vi "Handle Command.vi"(8 "error in (no error)":errorcluster, 10 "CMD in":refnum<class "Set Write Ringdowns CMD.lvclass">, 11 "Object In":refnum<class>) -> (0 "error out":errorcluster, 1 "Command Successful?":bool, 2 "CMD out":refnum<class "Set Write Ringdowns CMD.lvclass">, 3 "Object Out":refnum<class>)   [LabVIEW 2014, in "eCRDS Library.lvlib" / "Set Write Ringdowns CMD.lvclass"]
doc: "This VI will contain the code used to actually execute the request. If the request is successful, this will be indicated by the boolean output <b>Command Successful?</b>. The boolean output can then be used by the <b>Command Reply</b> which sends a reply if the reply queue is valid."
uses:
  Set Write Ringdowns CMD.lvclass
  reusable/CRDS/Main/CRDS.lvclass
  reusable/CRDS/Data/Main/CRDS Data.lvclass
  reusable/Instrument/Instrument.lvclass/Instrument.ctl
  Set Write Ringdowns CMD.lvclass/Set Write Ringdowns CMD.ctl
  reusable/CRDS/Cell/CRDS Cell.lvclass/CRDS Cell.ctl
  reusable/CRDS/Data/Cell/CRDS Cell Data.lvclass/CRDS Cell Data.ctl
  reusable/CRDS/Cell/Read Data.vi
  reusable/CRDS/Data/Cell/Write Write RD_.vi
  reusable/CRDS/Cell/Write Data.vi
  reusable/Instrument/Read Data.vi
  reusable/Instrument/Read Log Session.vi
  reusable/Instrument/Write Data.vi
  reusable/CRDS/Main/Read Cells.vi
  reusable/CRDS/Data/Main/Read CellData.vi
  reusable/CRDS/Data/Main/Write CellData.vi
  reusable/CRDS/Main/Write Cells.vi
  reusable/Data/Data.lvclass
  reusable/CRDS/Cell/CRDS Cell.lvclass
  <userlib>/_Session Fwk/Session - Root.lvclass
  reusable/CRDS/Data/Cell/CRDS Cell Data.lvclass
  reusable/Session APIs/Session Log/System Log.lvclass
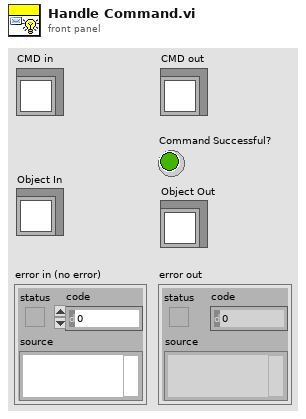
[diagram p1: front panel]
types:
  T1 = typedef "Session - Root.lvclass/Session Handle.ctl" = refnum<data-value>
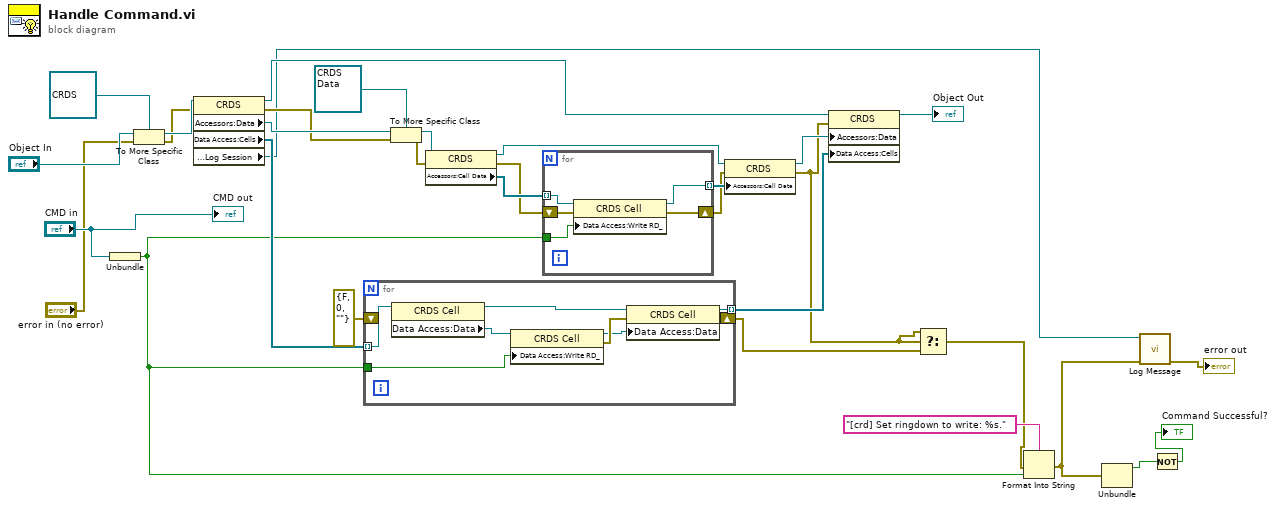
[diagram p0: block diagram]
diagram:
  n1 = Unbundle("CMD in") -> (w6:bool)
  n2 = To More Specific Class(target class=refnum<class "CRDS.lvclass"> refnum ("CRDS Lib.lvlib:CRDS"), reference="Object In", error in="error in (no error)") -> (specific class reference=w30:refnum<class "CRDS.lvclass">, error out=w16:errorcluster)
  n3 = property class="CRDS"(reference=w30, error in=w16) -> (reference out=w21:refnum<class "CRDS.lvclass">, error out=w15:errorcluster, "Accessors:Data"=w29:refnum<class "Data.lvclass">, "Data Access:Cells"=w24:refnum<class "CRDS Cell.lvclass">[], "Accessors:Log Session"=w8:T1)
  n4 = for {
    tunnel: w6 -> [w40]
    tunnel: w24 -> [w39] mode=indexing
    tunnel: [w34] -> w19 mode=indexing
    shift-right: [w33] -> w9
    shift-left: errorcluster {"status"=FALSE, "code"=0, "source"=""} ("error out") -> [_]
    n5 = property class="CRDS Cell"(reference=w39) -> (reference out=w36:refnum<class "CRDS Cell.lvclass">, "Data Access:Data"=w38:refnum<class "CRDS Cell Data.lvclass">)  [unwired: 1 in, 1 out]
    n6 = property class="CRDS Cell"(reference=w38, "Data Access:Write RD_"=w40) -> (reference out=w35:refnum<class "CRDS Cell Data.lvclass">, error out=w37:errorcluster)  [unwired: 1 in]
    n7 = property class="CRDS Cell"(reference=w36, error in=w37, "Data Access:Data"=w35) -> (reference out=w34:refnum<class "CRDS Cell.lvclass">, error out=w33:errorcluster)
  }
  n8 = To More Specific Class(target class=refnum<class "CRDS Data.lvclass"> refnum ("CRDS Lib.lvlib:CRDS"), reference=w29, error in=w15) -> (specific class reference=w27:refnum<class "CRDS Data.lvclass">, error out=w14:errorcluster)
  n9 = property class="CRDS"(reference=w27, error in=w14) -> (reference out=w22:refnum<class "CRDS Data.lvclass">, error out=w13:errorcluster, "Accessors:Cell Data"=w26:refnum<class "CRDS Cell Data.lvclass">[])
  n10 = for {
    tunnel: w26 -> [w45] mode=indexing
    tunnel: w6 -> [w44]
    tunnel: [w43] -> w23 mode=indexing
    shift-right: [w41] -> w12
    shift-left: w13 -> [w42]
    n11 = property class="CRDS Cell"(reference=w45, error in=w42, "Data Access:Write RD_"=w44) -> (reference out=w43:refnum<class "CRDS Cell Data.lvclass">, error out=w41:errorcluster)
  }
  n12 = property class="CRDS"(reference=w22, error in=w12, "Accessors:Cell Data"=w23) -> (reference out=w20:refnum<class "CRDS Data.lvclass">, error out=w10:errorcluster)
  n13 = property class="CRDS"(reference=w21, error in=w10, "Accessors:Data"=w20, "Data Access:Cells"=w19) -> (reference out=→"Object Out":refnum<class "CRDS.lvclass">)  [unwired: 1 out]
  n14 = Select(t=w10, s=w10, f=w9) -> (s? t:f=w5:errorcluster)
  n15 = Format Into String(format string="[crd] Set ringdown to write: %s.", error in=w5, w6) -> (error out=w4:errorcluster)  [unwired: 1 in, 1 out]
  n16 = Unbundle(w4) -> ("status"=w2:bool)  [unwired: 2 out]
  n17 = call "Log Message.vi"("error in"=w4, "session in"=w8) -> ("error out"=→"error out":errorcluster)  [unwired: 8 in, 1 out]
  n18 = Not(x=w2) -> (.not. x?=→"Command Successful?":bool)
  "CMD out" <- "CMD in"
